vi "Decode Number.vi"(8 "error in (no error)":errorcluster, 11 "json":string) -> (0 "error out":errorcluster, 2 "remaining json":string, 3 "value":variant)   [LabVIEW 2019, in "JSON.lvlib"]
doc: "Decodes JSON numbers: INT, UINT, DBL This supports extended numerics: +Inf, -Inf and NaN.\n\nCreated by: Ryan Pacini"
uses:
  JSON.lvlib
  <vilib>/regexp/Match Regular Expression.xnode
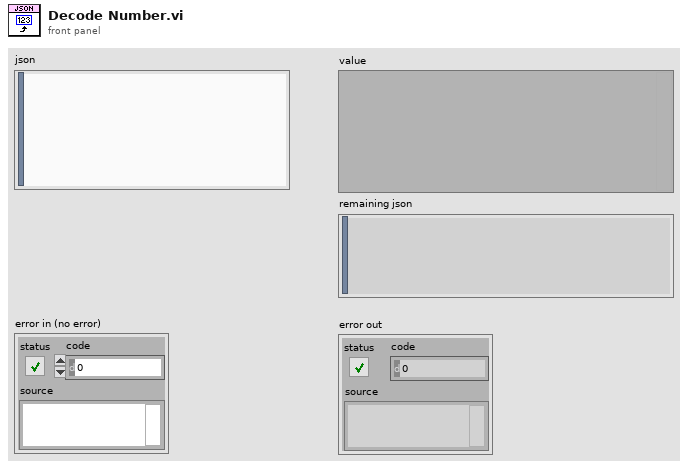
[diagram p1: front panel]
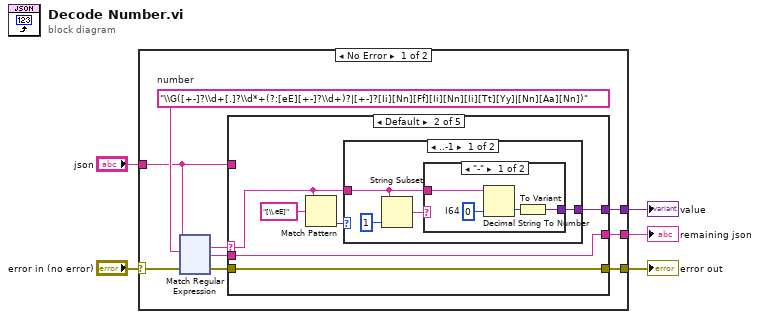
[diagram p0: block diagram]
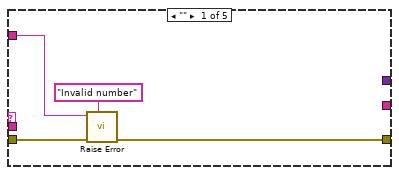
[diagram p2: hidden frame]
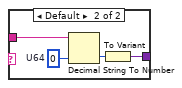
[diagram p3: hidden frame]
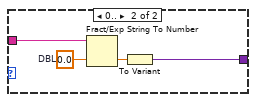
[diagram p4: hidden frame]
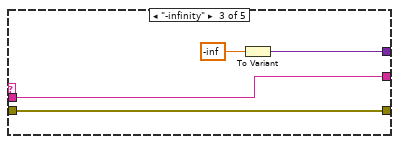
[diagram p5: hidden frame]
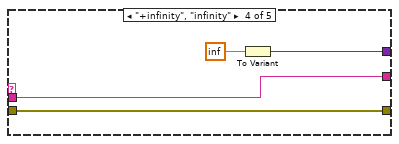
[diagram p6: hidden frame]
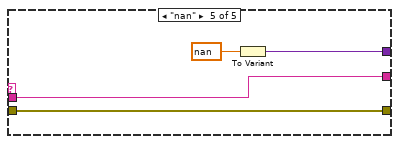
[diagram p7: hidden frame]
diagram:
  n1 = case shown="No Error" "error in (no error)" {
    selector: "error in (no error)" -> [w9 w167]
    tunnel: "json" -> [w10 _]
    tunnel: [w14 w167] -> w4
    tunnel: [w13 _] -> w2
    tunnel: [w7 _] -> w1
    frame No Error {
      w12 = "\\G([+-]?\\d+[.]?\\d*+(?:[eE][+-]?\\d+)?|[+-]?[Ii][Nn][Ff][Ii][Nn][Ii][Tt][Yy]|[Nn][Aa][Nn])"  # number
      n2 = xnode "Match Regular Expression"("input string"=w10, "regular expression"=w12, "error in"=w9) -> ("whole match"=w11:string, "after match"=w6:string, "error out"=w8:errorcluster)  [unwired: 3 in, 2 out]
      n3 = case shown="Default" w11 {
        selector: w11 -> [_ w136 _ _ _]
        tunnel: [w130 w134 w158 w162 w166] -> w14
        tunnel: w8 -> [w132 w134 w158 w162 w166]
        tunnel: [_ w135 w157 w161 w164] -> w13
        tunnel: w10 -> [w131 _ _ _ _]
        tunnel: [_ w133 w155 w159 w163] -> w7
        tunnel: w6 -> [_ w133 w155 w159 w163]
        frame "" {
          n4 = call "Raise Error.vi"("message"="Invalid number" ("error message (\"\")"), "error in (no error)"=w132, "json"=w131) -> ("error out"=w130:errorcluster)  [unwired: 8 in]
        }
        frame Default {
          n5 = Match Pattern(string=w136, regular expression="[\\.eE]") -> (offset past match=w137:i32)  [unwired: 1 in, 3 out]
          n6 = case shown="..-1" w137 {
            tunnel: w136 -> [w141 w154]
            tunnel: [w140 w151] -> w135
            frame ..-1 {
              n7 = String Subset(string=w141, length (rest)=1 ("length (rest)")) -> (substring=w139:string)  [unwired: 1 in]
              n8 = case shown="\"-\"" w139 {
                tunnel: w141 -> [w146 w150]
                tunnel: [w143 w147] -> w140
                frame "-" {
                  w145 = i64 0  # I64
                  n9 = Decimal String To Number(string=w146, default (0L)=w145) -> (number=w144:i64)  [unwired: 1 in, 1 out]
                  n10 = To Variant(anything=w144) -> (Variant=w143:variant)
                }
                frame Default {
                  w149 = u64 0  # U64
                  n11 = Decimal String To Number(string=w150, default (0L)=w149) -> (number=w148:u64)  [unwired: 1 in, 1 out]
                  n12 = To Variant(anything=w148) -> (Variant=w147:variant)
                }
              }
            }
            frame 0.. {
              w153 = 0.0  # DBL
              n13 = Fract/Exp String To Number(string=w154, default (0 dbl)=w153) -> (number=w152:dbl)  [unwired: 2 in, 1 out]
              n14 = To Variant(anything=w152) -> (Variant=w151:variant)
            }
          }
        }
        frame "-infinity" {
          n15 = To Variant(anything=-inf) -> (Variant=w157:variant)
        }
        frame "+infinity", "infinity" {
          n16 = To Variant(anything=inf) -> (Variant=w161:variant)
        }
        frame "nan" {
          n17 = To Variant(anything=nan) -> (Variant=w164:variant)
        }
      }
    }
    frame Error {
    }
  }
  "error out" <- w4
  "value" <- w2
  "remaining json" <- w1
